vi "ChangeWhileMeasuring.vi"(5 "StopOrRestart":enum16{"StopIfMeasuring", "RestartIfMeasuring"}(ring), 6 "WasMeasuring":bool, 7 "Queue Array In":refnum<queue>[](array[refnum]), 8 "error in (no error)":errorcluster, 11 "AcPwrBase in":refnum<class "AcPwrBase.lvclass">) -> (0 "error out":errorcluster, 3 "AcPwrBase out":refnum<class "AcPwrBase.lvclass">, 4 "WasMeasuring?":bool)   [LabVIEW 2018, in "AcPwrPlugins.lvlib" / "AcPwrBase.lvclass"]
doc: "This VI checks if the instrument is capable of send new instrument setting while the instruments is currently acquiring measurements."
uses:
  AcPwrBase.lvclass
  Common/clMessage.ctl
  AcPwrPlugins.lvlib
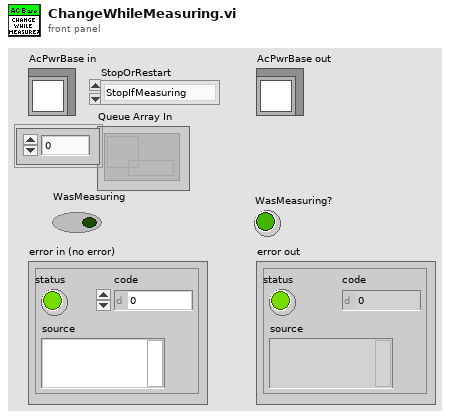
[diagram p1: front panel]
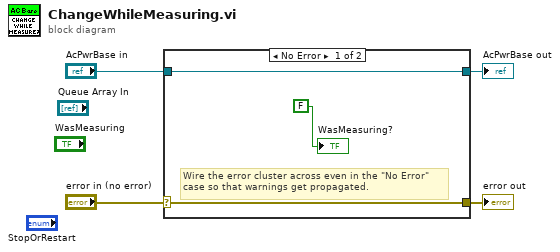
[diagram p0: block diagram]
diagram:
  n1 = case shown="No Error" "error in (no error)" {
    selector: "error in (no error)" -> [w6 w9]
    tunnel: [w6 w9] -> w3
    tunnel: [w7 w8] -> w1
    tunnel: "AcPwrBase in" -> [w7 w8]
    frame No Error {
      # "Wire the error cluster across even in the \"No Error\"\ncase so that warnings get propagated."
      "WasMeasuring?" <- FALSE ("OutputOrLoadState")
    }
    frame Error {
    }
  }
  "error out" <- w3
  "AcPwrBase out" <- w1
